vi "Double FFT Mesurament (Max Bin detection - Control - Windowing - Init Wave - Graph) test.vi"() -> ()   [LabVIEW 2014]
uses:
  <vilib>/Platform/TimedLoop/XDataNode/timing_clust.ctl
  <vilib>/Platform/TimedLoop/XDataNode/nitl_modes.ctl
  <vilib>/Platform/TimedLoop/XDataNode/wakeup.ctl
  <vilib>/rvi/Analysis/measure/FFT/simModelSupport/niFPGA FFT Streaming Sim Properties.ctl
  <vilib>/rvi/Analysis/measure/FFT/simModelSupport/niFPGA FFT Sim Stream Group Properties.ctl
  <vilib>/rvi/Analysis/measure/FFT/simModelSupport/niFPGA FFT Sim Types.ctl
  <vilib>/rvi/Analysis/measure/FFT/simModelSupport/niFpgaFFTSimArithmeticProperties.ctl
  <vilib>/rvi/Analysis/measure/FFT/simModelSupport/niFpgaFFTSimDfxp.ctl
  <vilib>/fxp/LVFixedPointQuantizationPolicyTypeDef.ctl
  <vilib>/rvi/Analysis/measure/FFT/XNode/niFpgaFFTButterflyDelays.ctl
  <vilib>/rvi/Emulation/niFpgaSctlEmulationGetInTimedLoop.vi
  <vilib>/rvi/Emulation/niFpgaEmulationReportErrorSimple.vi
  <vilib>/rvi/Emulation/niFpgaGetClockAttributes.vi
  <vilib>/rvi/Emulation/niFpgaCriticalErrorInLSC.vi
  <vilib>/rvi/Emulation/niFpgaEmulationIsFPGAContextNoSignature.vi
  <vilib>/rvi/errors/niFpgaSetErrorForExecOnDevCompSimple.vi
  <vilib>/rvi/eio/common/nirviEmuReportErrorAndStop.vi
  <vilib>/rvi/DataTransferAndStorage/Container/Common/niFpgaContainerGetUniqueNameForEmu.vi
  <vilib>/rvi/FIFO/Fifo_Resource/nirvififoEmulationSetSize.vi
  <vilib>/rvi/FIFO/Fifo_Resource/nirviFifoEmulationQueueMgr.vi
  <instcachedir>/0/nirviFifoEmulationQueueMgr_E5CAEC123FF24DC58D834DCA3CDAA9B5.lvgen/nirviFifoEmulationQueueMgr_E5CAEC123FF24DC58D834DCA3CDAA9B5_012.vi
  <vilib>/rvi/FIFO/Fifo_Resource/nirvififoEmulationCreateLock.vi
  <vilib>/rvi/Emulation/niFpgaProcessEmulError.vi
  <vilib>/rvi/FIFO/Fifo_Resource/nirvififoEmulationObtainLock.vi
  <vilib>/rvi/FIFO/Fifo_Resource/nirvififoEmulationReleaseLock.vi
  <vilib>/rvi/occurrence/nirviWaitOnOccurrenceBase.vi
  <vilib>/rvi/errors/nirviReportUnexpectedCaseInternalError.vi
  <vilib>/rvi/errors/nirviReportUnexpectedCaseInternalError (U32).vi
  <instcachedir>/0/nirviFifoEmulationQueueMgr_E5CAEC123FF24DC58D834DCA3CDAA9B5.lvgen/nirviFifoEmulationQueueMgr_E5CAEC123FF24DC58D834DCA3CDAA9B5_010.vi
  <vilib>/rvi/interface/RandomDataEmulation/niFpgaRandomDataHandleErrors.vi
  <vilib>/rvi/Memory/Memory_Emulation/niFpgaMemoryEmulationCacheClearOnFirstRun.vi
  <vilib>/rvi/Memory/Memory_Emulation/nirvimemoryEmulationManagerCache_MakeExclusive.vi
  <vilib>/rvi/Memory/Memory_Emulation/niFpgaMemoryEmulationValidateCache.vi
  <vilib>/rvi/Memory/Memory_Emulation/nirvimemoryEmulationManagerCache_InsertValue.vi
  <vilib>/Utility/error.llb/Clear Errors.vi
  <vilib>/rvi/Memory/Memory_Emulation/nirvimemoryEmulationManagerCache_ReleaseExclusive.vi
  <vilib>/rvi/Memory/Memory_Emulation/nirvimemoryEmulationManagerCache_GetValue.vi
  <vilib>/rvi/Memory/Memory_Emulation/nirvimemoryEmulationManagerCache_SetValue.vi
  <vilib>/rvi/FIFO/Fifo_Resource/nirvififoEmulationDetermineInputValidOut.vi
  <vilib>/rvi/Memory/Memory_Emulation/nirvimemoryFastEmulation.vi
  <vilib>/rvi/Memory/Memory_Emulation/nirvimemoryEmulation.vi
  <vilib>/rvi/Analysis/measure/FFT/simModelSupport/niFpgaFFTSimModelStreamingCore.vi
  <vilib>/rvi/eio/common/nirviEmuTemplateMethod_errors.vi
  <vilib>/Platform/TimedLoop/XDataNode/XDataNode.xnode
  <vilib>/rvi/DataTransferAndStorage/Container/XNode/niFpgaContainer.xnode
  <vilib>/rvi/FIFO/Fifo_Resource/nirvififoEmulationRead.vi
  <vilib>/rvi/interface/RandomDataEmulation/nirviRandomDataFpgaReadWriteTemplate.vi
  <vilib>/rvi/DataTransferAndStorage/Register/Emulation/niFpgaRegisterEmulation.vi
  <vilib>/rvi/FIFO/Fifo_Resource/nirvififoEmulationWrite.vi
  <vilib>/rvi/FIFO/Fifo_Resource/nirvififoEmulationGetNumberOfElementsToWrite.vi
  <vilib>/rvi/Analysis/measure/FFT/XNode/niFpgaFFT.xnode
  <vilib>/eio/EIOMethodNode/EIOMethodNode.xnode
  <vilib>/Platform/TimedLoop/XDataNode/XDNodeRunTimeDep.lvlib
panel:
  in  "snapshot":bool
  in  "first bin":i32=4
  in  "last bin":i32=251
  in  "lower limit 2":u32=682
  in  "lower limit 1":u32=57
  in  "upper limit 2":u32=1194
  in  "upper limit 1":u32=569
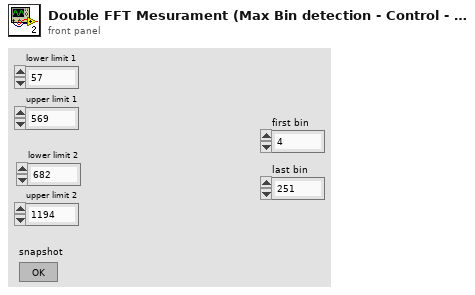
[diagram p1: front panel]
types:
  T1 = typedef "XDNodeRunTimeDep.lvlib/timing_clust.ctl" = cluster{"Expected End [f-1]":u64, "Actual End [f-1]":u64, "Finished Late? [f-1]":bool, "Expected End [i-1]":u64, "Actual End [i-1]":u64, "Finished Late? [i-1]":bool, "Expected Start [i]":u64, "Actual Start [i]":u64, "Expected Start [f]":u64, "Actual Start [f]":u64, "Source Name":string, "Structure Name":string, "Period":i64, "Deadline":i64, "Offset":i64, "Start":i64, "Priority":i32, "Timeout":i32, "Mode":T2, "Wakeup Reason":T3, "Error":errorcluster, "Source Type":string, "Secondary Source Type":string, "Global End Time":u64, "Global Start Time":u64, "Frame Duration":u64, "Iteration Duration":u64, "Assigned CPU":i32, "I/O Scan Engine Mode":u32}
  T2 = typedef "XDNodeRunTimeDep.lvlib/nitl_modes.ctl" = enum32{"No Change", "Process missed periods, maintain original phase", "Discard missed periods, maintain original phase", "Process missed periods, ignore original phase", "Discard missed periods, ignore original phase"}
  T3 = typedef "XDNodeRunTimeDep.lvlib/wakeup.ctl" = enum32{"Normal", "Aborted", "Asynchronous wakeup", "Timing source error", "Timed loop error", "Timeout"}
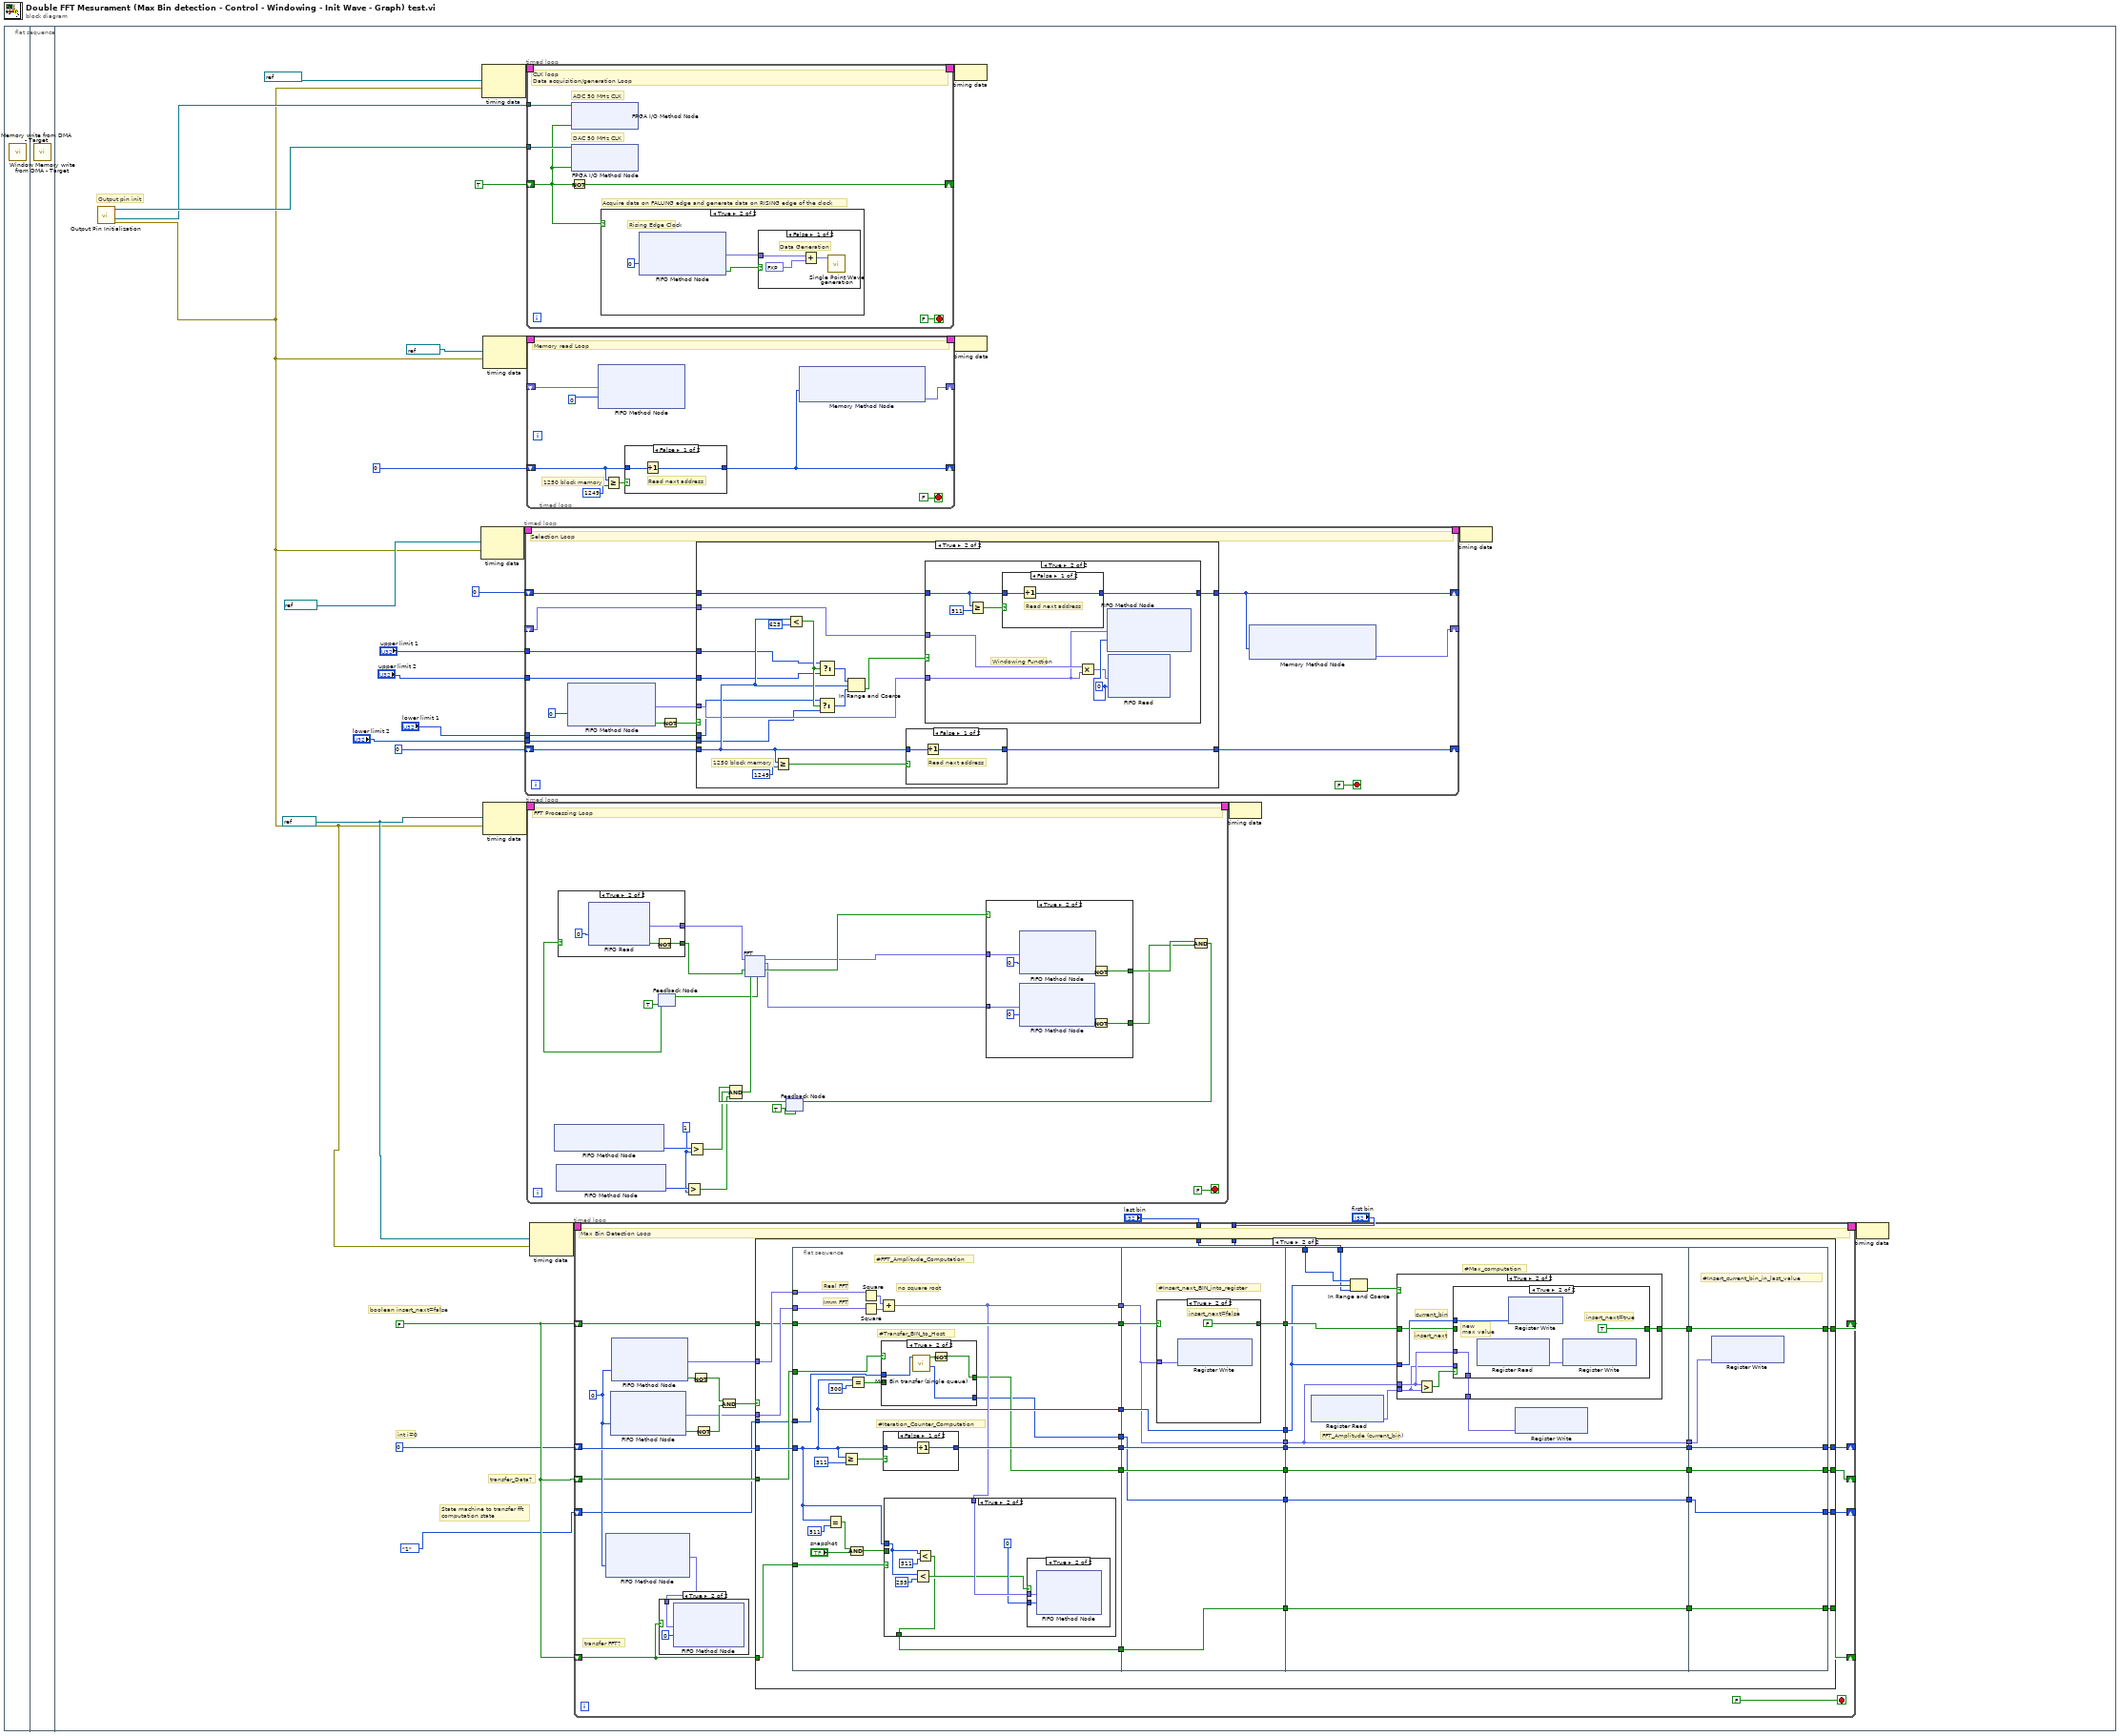
[diagram p0: block diagram]
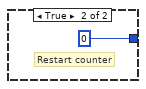
[diagram p7: hidden frame]
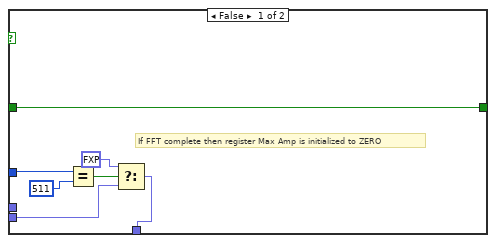
[diagram p9: hidden frame]
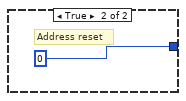
[diagram p13: hidden frame]
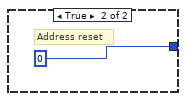
[diagram p14: hidden frame]
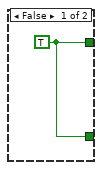
[diagram p15: hidden frame]
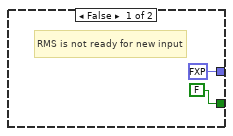
[diagram p16: hidden frame]
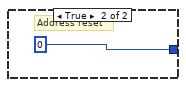
[diagram p17: hidden frame]
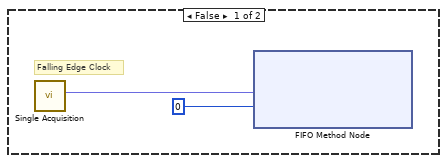
[diagram p18: hidden frame]
diagram:
  n1 = flat-sequence {
    frame #0 {
      n2 = call "Memory write from DMA - Target.vi"() -> ()  [unwired: 12 in]
    }
    frame #1 {
      n3 = call "Window Memory write from DMA - Target.vi"() -> ()  [unwired: 12 in]
    }
    frame #2 {
      w3 = FALSE
      w12 = refnum<k21> "50MHz" ("Source Name")
      # "State machine to transfer fft\ncomputation state"
      # "transfer_Data?"
      # "int i=0"
      # "boolean insert_next=false"
      # "Output pin init"
      n4 = call "Output Pin Initialization.vi"() -> ("error out"=w11:errorcluster, "I/O Out Clock DAC (pin16)"=w15:refnum<k21>, "I/O Out Clock ADC (pin17)"=w16:refnum<k21>)  [unwired: 8 in]
      n5 = node-c288(refnum<k21> "50MHz" ("Source Name"), w11) -> (w24:T1)
      n6 = node-c288(refnum<k21> "100MHz" ("Source Name"), w11) -> (w30:T1)
      n7 = node-c288(refnum<k21> "50MHz" ("Source Name"), w11) -> (w28:T1)
      n8 = node-c288(w12, w11) -> (w26:T1)
      n9 = timed-loop {
        timing: w24 -> [_]
        timing-out: [_] -> w23
        shift-right: [w205] -> _
        shift-left: u32 0 -> [w204]
        tunnel: "upper limit 1" -> [w199]
        tunnel: "upper limit 2" -> [w198]
        tunnel: "lower limit 1" -> [w197]
        tunnel: "lower limit 2" -> [w196]
        shift-right: [w192] -> _
        shift-left: u32 0 -> [w195]
        shift-right: [w193] -> _
        shift-left: _ -> [w194]
        stop <- FALSE stop-if-true
        # "Selection Loop"
        n10 = xnode ("FIFO Method Node")("Timeout"=0) -> ("Element"=w201:fxp<+/-,12,12>, "Timed Out?"=w202:bool)  [unwired: 1 in, 1 out]
        n11 = Not(x=w202) -> (.not. x?=w203:bool)
        n12 = case shown="True" w203 {
          tunnel: [w208 w223] -> w205
          tunnel: w204 -> [w208 w218]
          tunnel: w201 -> [_ w216]
          tunnel: w199 -> [_ w215]
          tunnel: w198 -> [_ w214]
          tunnel: w197 -> [_ w213]
          tunnel: w196 -> [_ w212]
          tunnel: w195 -> [w207 w209]
          tunnel: [w207 w211] -> w192
          tunnel: w194 -> [_ w210]
          frame False {
          }
          frame True {
            # "1250 block memory"
            n13 = Greater Or Equal?(x=w218, y=u32 1249) -> (x >= y?=w224:bool)
            n14 = Less?(x=w218, y=u32 625) -> (x < y?=w219:bool)
            n15 = Select(t=w213, s=w219, f=w212) -> (s? t:f=w221:u32)
            n16 = Select(t=w215, s=w219, f=w214) -> (s? t:f=w222:u32)
            n17 = In Range and Coerce(upper limit=w222, x=w218, lower limit=w221) -> (In Range?=w217:bool)  [unwired: 1 out]
            n18 = case shown="False" w224 {
              tunnel: w218 -> [w239 _]
              tunnel: [w238 u32 0] -> w223
              frame False {
                # "Read next address"
                n19 = Increment(x=w239) -> (x+1=w238:u32)
              }
              frame True {
                # "Address reset"
              }
            }
            n20 = case shown="True" w217 {
              tunnel: w216 -> [_ w227]
              tunnel: w209 -> [w226 w232]
              tunnel: [w226 w234] -> w211
              tunnel: w210 -> [_ w230]
              frame False {
              }
              frame True {
                w229 = 0 ("Timeout")
                # "Windowing Function"
                n21 = Greater Or Equal?(x=w232, y=u32 511) -> (x >= y?=w233:bool)
                n22 = case shown="False" w233 {
                  tunnel: w232 -> [w236 _]
                  tunnel: [w235 u32 0] -> w234
                  frame False {
                    # "Read next address"
                    n23 = Increment(x=w236) -> (x+1=w235:u32)
                  }
                  frame True {
                    # "Address reset"
                  }
                }
                n24 = Multiply(x=w230, y=w227) -> (x*y=w228:fxp<+/-,12,12>)
                n25 = xnode ("FIFO Method Node")("Element"=w227, "Timeout"=w229) -> ()  [unwired: 1 in, 2 out]
                n26 = xnode ("FIFO Read")("Element"=w228, "Timeout"=w229) -> ()  [unwired: 1 in, 2 out]
              }
            }
          }
        }
        n27 = xnode ("Memory Method Node")("Address"=w192) -> ("Data"=w193:fxp<+,8,1>)  [unwired: 1 in, 1 out]
      }
      n28 = timed-loop {
        timing: w30 -> [_]
        timing-out: [_] -> w29
        shift-right: [w336] -> _
        shift-left: TRUE -> [w334]
        tunnel: w15 -> [w338]
        tunnel: w16 -> [w335]
        stop <- FALSE stop-if-true
        # "DAC 50 MHz CLK"
        # "Acquire data on FALLING edge and generate data on RISING edge of the clock"
        # "ADC 50 MHz CLK"
        # "CLK loop\nData acquisition/generation Loop"
        n29 = Not(x=w334) -> (.not. x?=w336:bool)
        n30 = xnode "FPGA I/O Method Node"("FPGA I/O In"=w338, "Data"=w334) -> ()  [unwired: 1 out]
        n31 = xnode "FPGA I/O Method Node"("FPGA I/O In"=w335, "Data"=w334) -> ()  [unwired: 1 out]
        n32 = case shown="True" w334 {
          frame False {
            # "Falling Edge Clock"
            n33 = call "Single Acquisition.vi"() -> ("Out"=w340:fxp<+/-,12,12>)  [unwired: 10 in, 1 out]
            n34 = xnode ("FIFO Method Node")("Element"=w340, "Timeout"=0) -> ()  [unwired: 1 in, 2 out]
          }
          frame True {
            # "Rising Edge Clock"
            n35 = xnode ("FIFO Method Node")("Timeout"=0) -> ("Element"=w341:fxp<+/-,12,12>, "Timed Out?"=w342:bool)  [unwired: 1 in, 1 out]
            n36 = case shown="False" w342 {
              tunnel: w341 -> [w346 _]
              frame False {
                # "Data Generation"
                n37 = Add(x=w346, y=fxp<+,12,12> 2048.0) -> (x+y=w344:fxp<+/-,14,14>)
                n38 = call "Single Point Wave generation.vi"("Data To Write"=w344) -> ()  [unwired: 10 in, 1 out]
              }
              frame True {
                # "FPGA memory slow"
              }
            }
          }
        }
      }
      n39 = timed-loop {
        timing: w28 -> [_]
        timing-out: [_] -> w27
        shift-right: [w316] -> _
        shift-left: u32 0 -> [w320]
        shift-right: [w318] -> _
        shift-left: _ -> [w317]
        stop <- FALSE stop-if-true
        # "1250 block memory"
        # "Memory read Loop"
        n40 = xnode ("FIFO Method Node")("Element"=w317, "Timeout"=0) -> ()  [unwired: 1 in, 2 out]
        n41 = Greater Or Equal?(x=w320, y=u32 1249) -> (x >= y?=w322:bool)
        n42 = case shown="False" w322 {
          tunnel: w320 -> [w325 _]
          tunnel: [w324 u32 0] -> w316
          frame False {
            # "Read next address"
            n43 = Increment(x=w325) -> (x+1=w324:u32)
          }
          frame True {
            # "Address reset"
          }
        }
        n44 = xnode ("Memory Method Node")("Address"=w316) -> ("Data"=w318:fxp<+/-,12,12>)  [unwired: 1 in, 1 out]
      }
      n45 = timed-loop {
        timing: w26 -> [_]
        timing-out: [_] -> w25
        stop <- FALSE stop-if-true
        w250 = u32 1 ("y")
        # "FFT Processing Loop"
        n46 = xnode ("FIFO Method Node")() -> ("Number of Elements to Write"=w252:u32)  [unwired: 1 in, 1 out]
        n47 = xnode ("FIFO Method Node")() -> ("Number of Elements to Write"=w251:u32)  [unwired: 1 in, 1 out]
        n48 = feedback #1(TRUE ("ready for input")) -> (w267:bool)
        n49 = case shown="True" w267 {
          tunnel: [FALSE w308] -> w261
          tunnel: [fxp<+/-,12,12> 0.0 ("Element") w305] -> w262
          frame False {
            # "RMS is not ready for new input"
          }
          frame True {
            n50 = xnode ("FIFO Read")("Timeout"=0) -> ("Element"=w305:fxp<+/-,12,12>, "Timed Out?"=w307:bool)  [unwired: 1 in, 1 out]
            n51 = Not(x=w307) -> (.not. x?=w308:bool)
          }
        }
        n52 = Greater?(x=w251, y=w250) -> (0:w248:bool)
        n53 = Greater?(x=w252, y=w250) -> (0:w249:bool)
        n54 = feedback #2(TRUE) -> (w263:bool)
        n55 = Compound Arithmetic op=AND(w263, w249, w248) -> (w260:bool)
        n56 = xnode "FFT"("real data in"=w262, "input valid"=w261, "ready for output"=w260) -> ("ready for input"=w259:bool, "real data out"=w257:fxp<+/-,22,22>, "imaginary data out"=w256:fxp<+/-,22,22>, "output valid"=w258:bool)  [unwired: 2 in, 1 out]
        n57 = feedback-in #1(w259) -> ()
        n58 = case shown="True" w258 {
          tunnel: w257 -> [_ w302]
          tunnel: w256 -> [_ w301]
          tunnel: [w294 w300] -> w255
          tunnel: [w294 w299] -> w254
          frame False {
            w294 = TRUE
          }
          frame True {
            n59 = xnode ("FIFO Method Node")("Element"=w302, "Timeout"=0) -> ("Timed Out?"=w295:bool)  [unwired: 1 in, 1 out]
            n60 = xnode ("FIFO Method Node")("Element"=w301, "Timeout"=0) -> ("Timed Out?"=w296:bool)  [unwired: 1 in, 1 out]
            n61 = Not(x=w295) -> (.not. x?=w300:bool)
            n62 = Not(x=w296) -> (.not. x?=w299:bool)
          }
        }
        n63 = Compound Arithmetic op=AND(w255, w254) -> (w253:bool)
        n64 = feedback-in #2(w253) -> ()
      }
      n65 = node-c288(w12, w11) -> (w22:T1)
      n66 = timed-loop {
        shift-right: [w44] -> _
        shift-left: 0 ("Timeout") -> [w45]
        shift-right: [w42] -> _
        shift-left: w3 -> [w43]
        timing: w22 -> [_]
        timing-out: [_] -> w21
        tunnel: "last bin" -> [w40]
        tunnel: "first bin" -> [w39]
        shift-right: [w38] -> _
        shift-left: w3 -> [w32]
        shift-right: [w35] -> _
        shift-left: w3 -> [w36]
        shift-right: [w33] -> _
        shift-left: enum16{"1", "2", "3", "4"}."1" ("Enum") -> [w34]
        stop <- FALSE stop-if-true
        w37 = 0 ("Timeout")
        # "transfer FFT?"
        # "Max Bin Detection Loop"
        n67 = xnode ("FIFO Method Node")("Timeout"=w37) -> ("Element"=w31:fxp<+/-,12,12>)  [unwired: 1 in, 2 out]
        n68 = xnode ("FIFO Method Node")("Timeout"=w37) -> ("Element"=w46:fxp<+/-,22,22>, "Timed Out?"=w51:bool)  [unwired: 1 in, 1 out]
        n69 = xnode ("FIFO Method Node")("Timeout"=w37) -> ("Element"=w47:fxp<+/-,22,22>, "Timed Out?"=w52:bool)  [unwired: 1 in, 1 out]
        n70 = case shown="True" w32 {
          tunnel: w31 -> [_ w54]
          frame False {
          }
          frame True {
            n71 = xnode ("FIFO Method Node")("Element"=w54, "Timeout"=0) -> ()  [unwired: 1 in, 2 out]
          }
        }
        n72 = Not(x=w52) -> (.not. x?=w50:bool)
        n73 = Not(x=w51) -> (.not. x?=w49:bool)
        n74 = And(x=w50, y=w49) -> (x .and. y?=w48:bool)
        n75 = case shown="True" w48 {
          tunnel: w47 -> [_ w93]
          tunnel: w46 -> [_ w92]
          tunnel: w45 -> [w59 w90]
          tunnel: [w59 w77] -> w44
          tunnel: w43 -> [w58 w84]
          tunnel: [w58 w79] -> w42
          tunnel: w40 -> [_ w76]
          tunnel: w39 -> [_ w75]
          tunnel: [w57 w71] -> w38
          tunnel: w32 -> [w57 w70]
          tunnel: w36 -> [w56 w69]
          tunnel: [w56 w68] -> w35
          tunnel: w34 -> [w55 w64]
          tunnel: [w55 w60] -> w33
          frame False {
            # "Data are NOT ready in Target Real FFT and Target Imm FFT FIFOs"
          }
          frame True {
            n76 = flat-sequence {
              tunnel: w93 -> [w112]
              tunnel: w92 -> [w113]
              tunnel: [w103] -> w91
              tunnel: w90 -> [w99]
              tunnel: [w111] -> w89
              tunnel: [w99] -> w86
              tunnel: [w108] -> w85
              tunnel: w84 -> [w108]
              tunnel: [w101] -> w74
              tunnel: w70 -> [w100]
              tunnel: w69 -> [w98]
              tunnel: [w96] -> w67
              tunnel: w64 -> [w95]
              tunnel: [w94] -> w61
              tunnel: w91 -> [w139]
              tunnel: w89 -> [w142]
              tunnel: [w142] -> w88
              tunnel: w86 -> [w140]
              tunnel: w85 -> [w141]
              tunnel: [w140] -> w83
              tunnel: [w139] -> w82
              tunnel: [w138] -> w81
              tunnel: w74 -> [w137]
              tunnel: [w137] -> w72
              tunnel: w67 -> [w136]
              tunnel: [w136] -> w66
              tunnel: [w135] -> w62
              tunnel: w61 -> [w135]
              tunnel: w88 -> [w158]
              tunnel: [w158] -> w87
              tunnel: w83 -> [w153]
              tunnel: w82 -> [w155]
              tunnel: w81 -> [w156]
              tunnel: [w155] -> w80
              tunnel: [w154] -> w78
              tunnel: w76 -> [w150]
              tunnel: w75 -> [w149]
              tunnel: [w148] -> w73
              tunnel: w72 -> [w148]
              tunnel: w66 -> [w147]
              tunnel: [w147] -> w65
              tunnel: [w146] -> w63
              tunnel: w62 -> [w146]
              tunnel: w87 -> [w182]
              tunnel: w80 -> [w184]
              tunnel: w78 -> [w183]
              tunnel: [w183] -> w79
              tunnel: [w182] -> w77
              tunnel: [w181] -> w71
              tunnel: w73 -> [w181]
              tunnel: [w180] -> w68
              tunnel: w65 -> [w180]
              tunnel: w63 -> [w179]
              tunnel: [w179] -> w60
              frame #0 {
                # "no square root"
                # "#Transfer_BIN_to_Host"
                # "#Iteration_Counter_Computation"
                # "#FFT_Amplitude_Computation"
                # "Imm FFT"
                # "Real FFT"
                n77 = Equal?(x=w99, y=511) -> (x = y?=w104:bool)
                n78 = Greater Or Equal?(x=w99, y=511) -> (x >= y?=w109:bool)
                n79 = Equal?(x=w99, y=300) -> (x = y?=w97:bool)
                n80 = Compound Arithmetic op=AND(w104, "snapshot") -> (w102:bool)
                n81 = Square(x=w112) -> (x^2=w115:fxp<+,43,43>)
                n82 = Square(x=w113) -> (x^2=w114:fxp<+,43,43>)
                n83 = Add(x=w115, y=w114) -> (x+y=w103:fxp<+,44,44>)
                n84 = case shown="True" w98 {
                  tunnel: w97 -> [w127 _]
                  tunnel: [w127 w130] -> w96
                  tunnel: w95 -> [w126 w129]
                  tunnel: [w126 w128] -> w94
                  frame False {
                    # "FFT Comp is NOT finished"
                  }
                  frame True {
                    n85 = call "Max Bin transfer (single queue).vi"("Enum"=w129) -> ("Next state"=w128:enum16{"1", "2", "3", "4"}, "END?"=w131:bool)  [unwired: 9 in]
                    n86 = Not(x=w131) -> (.not. x?=w130:bool)
                  }
                }
                n87 = case shown="False" w109 {
                  tunnel: w99 -> [w132 _]
                  tunnel: [w133 0 ("Timeout")] -> w111
                  frame False {
                    n88 = Increment(x=w132) -> (x+1=w133:i32)
                  }
                  frame True {
                    # "Restart counter"
                  }
                }
                n89 = case shown="True" w100 {
                  tunnel: w103 -> [_ w123]
                  tunnel: w102 -> [w116 _]
                  tunnel: [w116 w117] -> w101
                  tunnel: w99 -> [_ w118]
                  frame False {
                  }
                  frame True {
                    n90 = Less?(x=w118, y=255) -> (x < y?=w120:bool)
                    n91 = Less?(x=w118, y=511) -> (x < y?=w117:bool)
                    n92 = case shown="True" w120 {
                      tunnel: w123 -> [_ w125]
                      tunnel: 0 ("Timeout") -> [_ w124]
                      frame False {
                      }
                      frame True {
                        n93 = xnode ("FIFO Method Node")("Element"=w125, "Timeout"=w124) -> ()  [unwired: 1 in, 2 out]
                      }
                    }
                  }
                }
              }
              frame #1 {
                # "#Insert_next_BIN_into_register"
                n94 = case shown="True" w141 {
                  selector: w141 -> [w143 _]
                  tunnel: [w143 FALSE] -> w138
                  tunnel: w139 -> [_ w144]
                  frame False {
                  }
                  frame True {
                    # "insert_next=false"
                    n95 = xnode ("Register Write")("Data"=w144) -> ()  [unwired: 1 in, 1 out]
                  }
                }
              }
              frame #2 {
                # "FFT_Amplitude (current_bin)"
                # "#Max_computation"
                n96 = xnode ("Register Read")() -> ("Data"=w152:fxp<+,44,44>)  [unwired: 1 in, 1 out]
                n97 = In Range and Coerce(upper limit=w150, x=w153, lower limit=w149) -> (In Range?=w157:bool)  [unwired: 1 out]
                n98 = case shown="True" w157 {
                  tunnel: w155 -> [_ w171]
                  tunnel: w153 -> [w163 w170]
                  tunnel: w156 -> [w165 w169]
                  tunnel: [w165 w168] -> w154
                  tunnel: w152 -> [w161 w166]
                  tunnel: [w159 w167] -> w151
                  frame False {
                    # "If FFT complete then register Max Amp is initialized to ZERO"
                    n99 = Equal?(x=w163, y=511) -> (x = y?=w164:bool)
                    n100 = Select(t=fxp<+,44,44> 0.0, s=w164, f=w161) -> (s? t:f=w159:fxp<+,44,44>)
                  }
                  frame True {
                    # "insert_next"
                    # "current_bin"
                    n101 = Greater?(x=w171, y=w166) -> (0:w172:bool)
                    n102 = case shown="True" w172 {
                      tunnel: w171 -> [_ w175]
                      tunnel: w170 -> [_ w178]
                      tunnel: w169 -> [w174 _]
                      tunnel: [w174 TRUE] -> w168
                      tunnel: [w173 w175] -> w167
                      tunnel: w166 -> [w173 _]
                      frame False {
                        # "Old value is re-written"
                      }
                      frame True {
                        # "new\nmax value"
                        # "insert_next=true"
                        n103 = xnode ("Register Read")() -> ("Data"=w176:fxp<+,44,44>)  [unwired: 1 in, 1 out]
                        n104 = xnode ("Register Write")("Data"=w178) -> ()  [unwired: 1 in, 1 out]
                        n105 = xnode ("Register Write")("Data"=w176) -> ()  [unwired: 1 in, 1 out]
                      }
                    }
                  }
                }
                n106 = xnode ("Register Write")("Data"=w151) -> ()  [unwired: 1 in, 1 out]
              }
              frame #3 {
                # "#Insert_current_bin_in_last_value"
                n107 = xnode ("Register Write")("Data"=w184) -> ()  [unwired: 1 in, 1 out]
              }
            }
          }
        }
      }
      n108 = node-c288(w29) -> ()
      n109 = node-c288(w27) -> ()
      n110 = node-c288(w25) -> ()
      n111 = node-c288(w23) -> ()
      n112 = node-c288(w21) -> ()
    }
  }
